vi "check.vi"(8 "error in (no error)":errorcluster) -> (0 "error out":errorcluster)   [LabVIEW 2015, in "lv-config-json.lvlib"]
doc: "This VI will check to see if the configuration exists, if it does exist, it doesn't do anything. If it doesn't exist, it will copy the default configuration from the data folder to the working directory for configuration."
uses:
  lv-config-json.lvlib
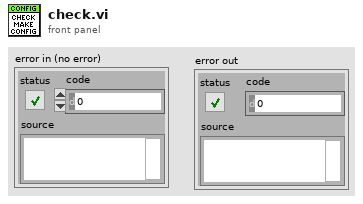
[diagram p1: front panel]
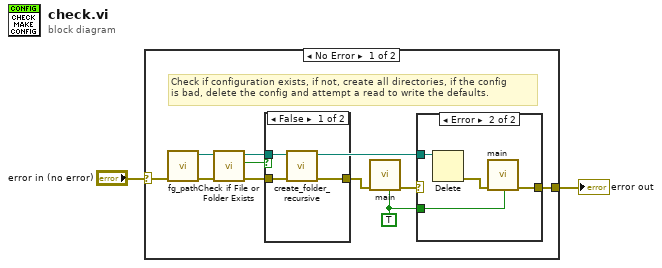
[diagram p0: block diagram]
diagram:
  n1 = case shown="No Error" "error in (no error)" {
    selector: "error in (no error)" -> [w12 w22]
    tunnel: [w4 w22] -> w2
    frame No Error {
      w3 = TRUE ("force_read?")
      # "Check if configuration exists, if not, create all directories, if the config\nis bad, delete the config and attempt a read to write the defaults."
      n2 = call "fg_path.vi"("error in (no error)"=w12) -> ("error out"=w10:errorcluster, "config_working"=w11:path)  [unwired: 9 in]
      n3 = call <vilib>:"Check if File or Folder Exists.vi"("error in (no error)"=w10, "path"=w11) -> ("error out"=w9:errorcluster, "file or folder exists?"=w8:bool, "dup path"=w5:path)  [unwired: 7 in]
      n4 = case shown="False" w8 {
        tunnel: w5 -> [w20 _]
        tunnel: w9 -> [w19 w21]
        tunnel: [w18 w21] -> w6
        frame False {
          n5 = call "create_folder_recursive.vi"("error in"=w19, "path in"=w20) -> ("error out"=w18:errorcluster)  [unwired: 8 in, 1 out]
        }
        frame True {
        }
      }
      n6 = call "main.vi"("force_read?"=w3, "error in (no error)"=w6) -> ("error out"=w7:errorcluster)  [unwired: 8 in, 1 out]
      n7 = case shown="Error" w7 {
        selector: w7 -> [w13 _]
        tunnel: w5 -> [_ w17]
        tunnel: [w13 w15] -> w4
        tunnel: w3 -> [_ w14]
        frame No Error {
        }
        frame Error {
          n8 = Delete(path (use dialog)=w17) -> (error out=w16:errorcluster)  [unwired: 4 in, 2 out]
          n9 = call "main.vi"("force_read?"=w14, "error in (no error)"=w16) -> ("error out"=w15:errorcluster)  [unwired: 8 in, 1 out]
        }
      }
    }
    frame Error {
    }
  }
  "error out" <- w2
